vi "FULL ADDER.vi"(2 "C":bool, 3 "B":bool, 4 "A":bool) -> (0 "CARRY":bool, 1 "SUM":bool)   [LabVIEW 2017]
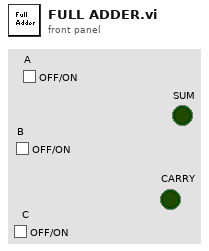
[diagram p1: front panel]
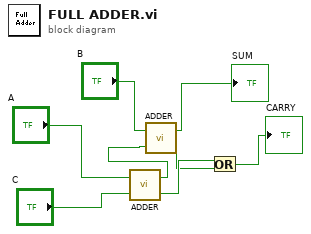
[diagram p0: block diagram]
diagram:
  n1 = call "ADDER.vi"("INPUT2"="C", "INPUT1"="A") -> ("CARRY"=w6:bool, "SUM"=w1:bool)
  n2 = call "ADDER.vi"("INPUT2"=w1, "INPUT1"="B") -> ("CARRY"=w4:bool, "SUM"=→"SUM":bool)
  n3 = Or(x=w6, y=w4) -> (x .or. y?=→"CARRY":bool)
